vi "helper-log-parse-auxi.vi"(10 "log cluster":T2 {"clk" format="%#.3f"}, 11 "AuxiliaryList in":T1(array[cluster])) -> (3 "AuxiliaryList out":T1(array[cluster]))   [LabVIEW 2024]
uses:
  controls/typeEngineLogCluster.ctl
  controls/type.StepFunction.ctl
panel:
  out "error IO":errorcluster
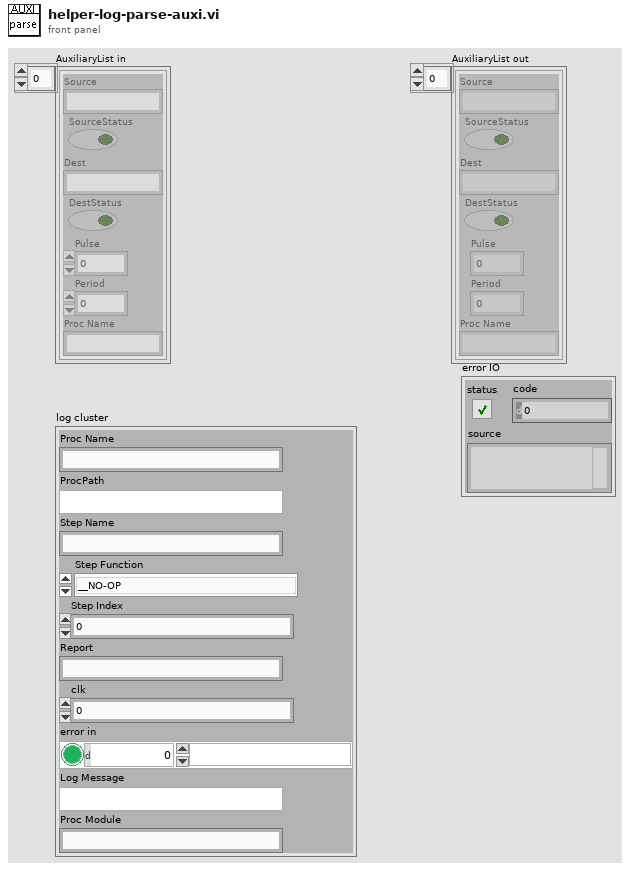
[diagram p1: front panel]
types:
  T1 = cluster{"Source":string, "SourceStatus":bool, "Dest":string, "DestStatus":bool, "Pulse":u16, "Period":u16, "Proc Name":string}[]
  T2 = typedef "typeEngineLogCluster.ctl" = cluster{"Proc Name":string, "ProcPath":string, "Step Name":string, "Step Function":T3, "Step Index":i32, "Report":string, "clk":dbl, "error in":errorcluster, "Log Message":string, "Proc Module":string}
  T3 = typedef "type.StepFunction.ctl" = enum16{"__NO-OP", "_DELAY_LOAD", "_DELAY_COMPARE", "_JUMP", "_COMPLETE", "_COMPARE", "_LOG_MESSAGE", "_LOG_LAST_REPORT", "_SCHEDULE", "_SCHED_DAILY", "CLK_COMPARE", "PROC_START", "PROC_STOP", "PROC_LOAD", "PROC_COMPLETION_CHECK", "PROC_COMPLETION_LOAD", "_IO_READ", "_IO_READ_MANY", "_IO_WRITE", "_IO_WRITE_BY_REG", "_IO_GET_OUTPUT", "_OCS_CHECK", "_OCS_RECORD", "_GET_RH", "_GET_ACC_UV", "_GET_WD", "_GET_WS", "_REC_DELETE", "_REC_MOVE", "_REC_COPY", "_IRR_CHECK", "UNIT_CHECK", "UNIT_SAMPLE", "UNIT_DOSE"}
  T4 = cluster{"Source":string, "SourceStatus":bool, "Dest":string, "DestStatus":bool, "Pulse":u16, "Period":u16, "Proc Name":string}
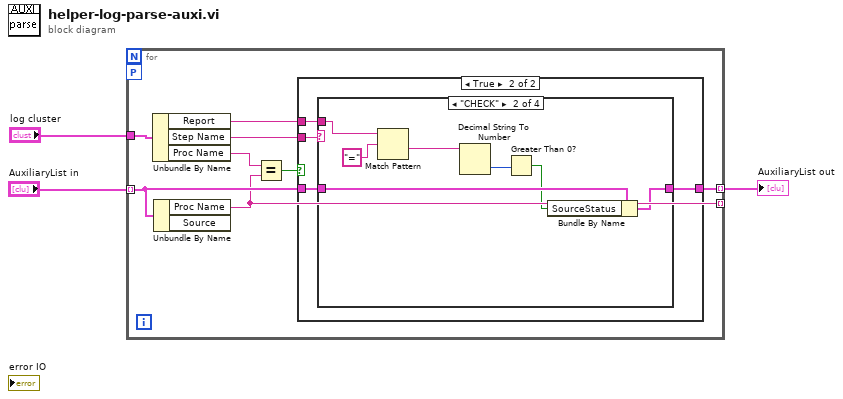
[diagram p0: block diagram]
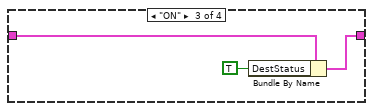
[diagram p4: hidden frame]
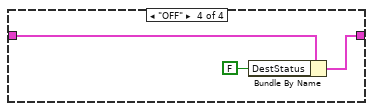
[diagram p5: hidden frame]
diagram:
  n1 = for {
    tunnel: "AuxiliaryList in" -> [w11] mode=indexing
    tunnel: [w10] -> w1 mode=indexing
    tunnel: "log cluster" -> [w9]
    tunnel: [w4] -> _ mode=indexing
    workers-P: _ -> [_]
    n2 = Unbundle By Name(w9) -> ("Report"=w8:string, "Step Name"=w6:string, "Proc Name"=w7:string)
    n3 = Unbundle By Name(w11) -> ("Proc Name"=w4:string)  [unwired: 1 out]
    n4 = Equal?(x=w7, y=w4) -> (x = y?=w5:bool)
    n5 = case shown="True" w5 {
      tunnel: w11 -> [w12 w16]
      tunnel: [w12 w15] -> w10
      tunnel: w8 -> [_ w14]
      tunnel: w6 -> [_ w13]
      frame False {
      }
      frame True {
        n6 = case shown="\"CHECK\"" w13 {
          tunnel: w16 -> [w17 w24 w27 w30]
          tunnel: [w17 w23 w26 w29] -> w15
          tunnel: w14 -> [_ w22 _ _]
          frame Default {
          }
          frame "CHECK" {
            n7 = Match Pattern(string=w22, regular expression="=") -> (after substring=w20:string)  [unwired: 1 in, 3 out]
            n8 = Decimal String To Number(string=w20) -> (number=w19:i32)  [unwired: 2 in, 1 out]
            n9 = Greater Than 0?(x=w19) -> (x > 0?=w18:bool)
            n10 = Bundle By Name(cluster=w24, "SourceStatus"=w18) -> (w23:T4)
          }
          frame "ON" {
            n11 = Bundle By Name(cluster=w27, "DestStatus"=TRUE ("SourceStatus")) -> (w26:T4)
          }
          frame "OFF" {
            n12 = Bundle By Name(cluster=w30, "DestStatus"=FALSE ("SourceStatus")) -> (w29:T4)
          }
        }
      }
    }
  }
  "AuxiliaryList out" <- w1
